vi "WiiMote Open.vi"() -> (0 "error out":errorcluster, 3 "WiiMote reference":refnum<k24>)   [LabVIEW 2013]
uses:
  D:/Users/jjensen/Documents/Lab Book/embeddedLab/exercises/LabVIEW/WiiMote/Dependencies/WiimoteLib.dll
  Dependencies/WiimoteLib.dll
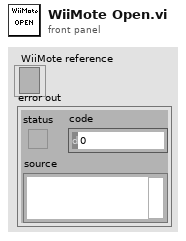
[diagram p1: front panel]
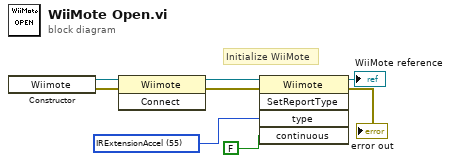
[diagram p0: block diagram]
diagram:
  w6 = u8 55 items=["Status"=32, "ReadData"=33, "OutputReportAck"=34, "Buttons"=48, "ButtonsAccel"=49, "IRAccel"=51, "ButtonsExtension"=52, "ExtensionAccel"=53, "IRExtensionAccel"=55] ("type")
  # "Initialize WiiMote"
  n1 = constructor class="Wiimote"() -> (reference out=w7:refnum<k24>, error out=w8:errorcluster)  [unwired: 3 in, 1 out]
  n2 = invoke class="Wiimote" method="Connect"(reference=w7, error in=w8) -> (reference out=w3:refnum<k24>, error out=w5:errorcluster)  [unwired: 1 in, 1 out]
  n3 = invoke class="Wiimote" method="SetReportType"(reference=w3, error in=w5, "type"=w6, "continuous"=FALSE) -> (reference out=→"WiiMote reference":refnum<k24>, error out=→"error out":errorcluster)  [unwired: 1 in, 3 out]
